vi "Get Transfer Group Status.vi"(11 "Framework Status in":refnum<class "Framework Status.lvclass">) -> (2 "Transfer Group Status":refnum<class "Transfer Group Status.lvclass">, 3 "Framework Status out":refnum<class "Framework Status.lvclass">)   [LabVIEW 2017, in "DSF Core.lvlib" / "Framework Status.lvclass"]
uses:
  Status/Framework Status.lvclass
  Transfer Group Status/Transfer Group Status.lvclass
  Status/Framework Status.lvclass/Framework Status.ctl
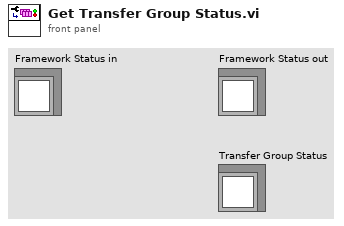
[diagram p1: front panel]
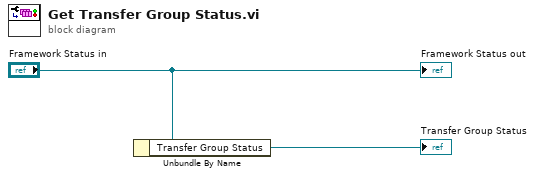
[diagram p0: block diagram]
diagram:
  n1 = Unbundle By Name("Framework Status in") -> ("Transfer Group Status"=→"Transfer Group Status":refnum<class "Transfer Group Status.lvclass">)
  "Framework Status out" <- "Framework Status in"
